vi "SolenoidSwitch.vi"(0 "RefNum Name":string="My Solenoid RefNum", 1 "Button":bool) -> (2 "Solenoid Value":T1, 3 "Solenoid Bool":bool, 4 "Solenoid State":i32(knob) scale=0.0..4.0)   [LabVIEW 2017]
uses:
  <vilib>/Rock Robotics/WPI/Solenoid/WPI_SolenoidValue.ctl
  <vilib>/Rock Robotics/WPI/Solenoid/WPI_SolenoidSetEnum.vi
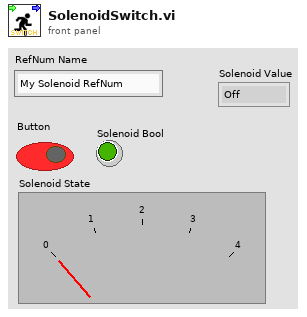
[diagram p1: front panel]
types:
  T1 = typedef "WPI_SolenoidValue.ctl" = enum16{"Off", "On", "Forward", "Reverse"}
  T2 = typedef "WPI_SolenoidDevRef.ctl" = cluster{"DevStatus":errorcluster, "Pneumatics Control Module":u8, "Forward Solenoid Channel":T3, "Reverse Solenoid Channel":T3}
  T3 = typedef "WPI_SolenoidChannel.ctl" = enum8{"Solenoid 0", "Solenoid 1", "Solenoid 2", "Solenoid 3", "Solenoid 4", "Solenoid 5", "Solenoid 6", "Solenoid 7", "Invalid"}
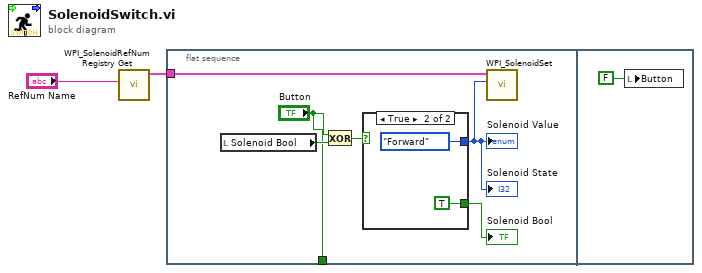
[diagram p0: block diagram]
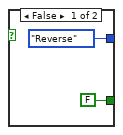
[diagram p2: hidden frame]
diagram:
  n1 = call <vilib>:"WPI_SolenoidRefNum Registry Get.vi"("refnum name"="RefNum Name") -> ("SolenoidDevRef"=w1:T2)  [unwired: 9 in, 1 out]
  n2 = flat-sequence {
    tunnel: ["Button"] -> _
    tunnel: w1 -> [w4]
    frame #0 {
      n3 = local read "Solenoid Bool"() -> (w6:bool)
      n4 = Exclusive Or(1:w6, 2:"Button") -> (0:w7:bool)
      n5 = case shown="True" w7 {
        tunnel: [FALSE TRUE] -> w8
        tunnel: [WPI_SolenoidValue."Reverse" ("Value") WPI_SolenoidValue."Forward" ("Value")] -> w3
        frame False {
        }
        frame True {
        }
      }
      "Solenoid Bool" <- w8
      "Solenoid State" <- w3
      "Solenoid Value" <- w3
      n6 = call-poly <vilib>:"WPI_SolenoidSet.vi"("Value"=w3, "SolenoidDevRef"=w4) -> ()  [unwired: 8 in, 2 out]
    }
    frame #1 {
      n7 = local write "Button"(FALSE ("BoolIn")) -> ()
    }
  }
